vi "get NormName.vi"(8 "error in (no error)":errorcluster caption="Fehler (Eingang, kein Fehler)", 11 "Test (Eingang)":refnum<class "Norm.lvclass">) -> (0 "error out":errorcluster caption="Fehler (Ausgang)", 2 "name":string, 3 "Test (Ausgang)":refnum<class "Norm.lvclass">)   [LabVIEW 2013, in "DatenKlassen.lvlib" / "Norm.lvclass"]
uses:
  Norm.lvclass
  Norm.lvclass/Norm.ctl
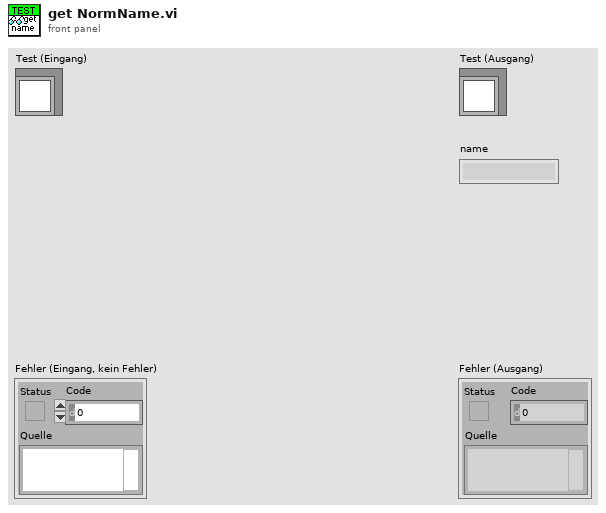
[diagram p1: front panel]
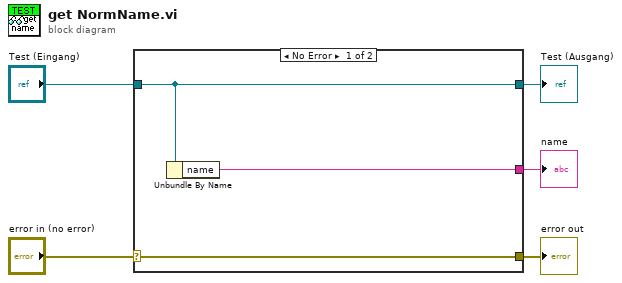
[diagram p0: block diagram]
diagram:
  n1 = case shown="No Error" "error in (no error)" {
    selector: "error in (no error)" -> [w8 w9]
    tunnel: [w8 w9] -> w4
    tunnel: [w7 w10] -> w2
    tunnel: "Test (Eingang)" -> [w7 w10]
    tunnel: [w6 _] -> w1
    frame No Error {
      n2 = Unbundle By Name(w7) -> ("name"=w6:string)
    }
    frame Error {
    }
  }
  "error out" <- w4
  "Test (Ausgang)" <- w2
  "name" <- w1
